vi "Change Administrator Password.vi"(8 "error in (no error)":errorcluster, 10 "New Password":string, 11 "Session in":refnum<k21>="localhost") -> (0 "error out":errorcluster, 3 "Session out":refnum<k21>)   [LabVIEW 2017, in "nisyscfg.lvlib"]
doc: "Change the administrator password. This requires Secure Shell Server (sshd) to be enabled on the target."
uses:
  <vilib>/nisyscfg/nisyscfg.lvlib
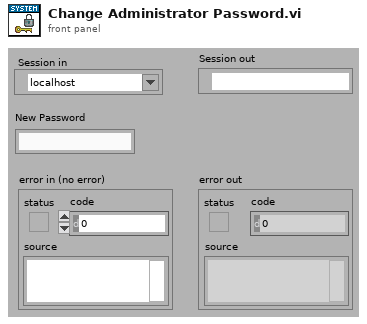
[diagram p1: front panel]
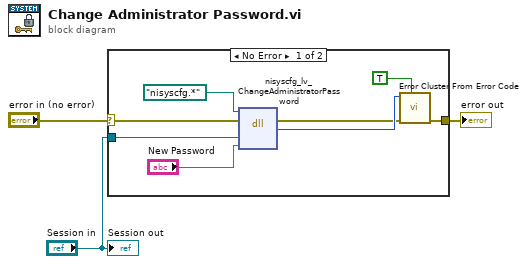
[diagram p0: block diagram]
diagram:
  n1 = case shown="No Error" "error in (no error)" {
    selector: "error in (no error)" -> [w8 w12]
    tunnel: [w11 w12] -> w3
    tunnel: "Session in" -> [w7 _]
    frame No Error {
      n2 = dll-call lib="nisyscfg.*" fn="nisyscfg_lv_ChangeAdministratorPassword" label="ChangeAdministratorPassword"(path in=path "nisyscfg.*", error in=w8, "sessionHandle"=w7, "newPassword"="New Password") -> (error out=w9:errorcluster, "return type"=w10:i32)  [unwired: 3 in, 1 out]
      n3 = call <vilib>:"Error Cluster From Error Code.vi"("show call chain? (False)"=TRUE, "error in (no error)"=w9, "error code (0)"=w10) -> ("error out"=w11:errorcluster)  [unwired: 6 out]
    }
    frame Error {
    }
  }
  "error out" <- w3
  "Session out" <- "Session in"
